vi "Compute Complementary Amplitude Multi-Exponential.vi"(8 "Error In":errorcluster, 9 "Time Constant Array":dbl[](array[numeric]), 11 "Amplitude Array":dbl[](array[numeric])) -> (0 "Error Out":errorcluster, 3 "Complementary Amplitude":dbl)   [LabVIEW 2021, in "Fits.lvlib"]
uses:
  Fits.lvlib
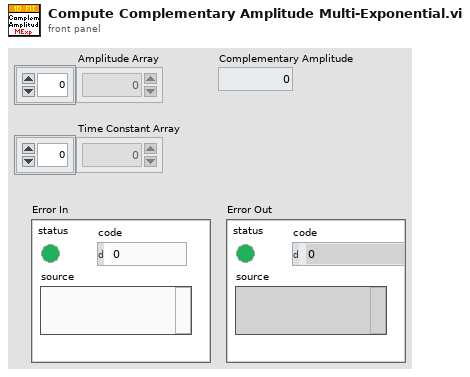
[diagram p1: front panel]
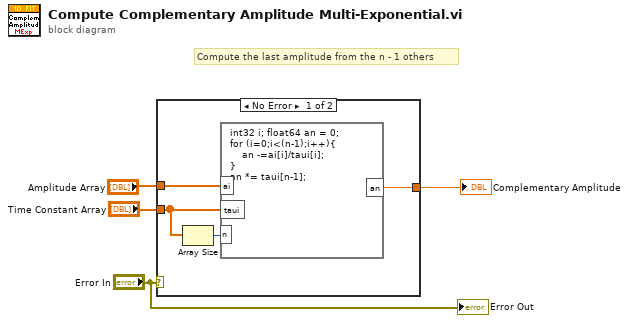
[diagram p0: block diagram]
diagram:
  # "Compute the last amplitude from the n - 1 others"
  n1 = case shown="No Error" "Error In" {
    tunnel: [w8 _] -> w4
    tunnel: "Amplitude Array" -> [w7 _]
    tunnel: "Time Constant Array" -> [w6 _]
    frame No Error {
      n2 = Array Size(array=w6) -> (size(s)=w5:i32)
      n3 = formula code="int32 i; float64 an = 0; \nfor (i=0;i<(n-1);i++){\n    an -=ai[i]/taui[i];\n}\nan *= taui[n-1];"("ai"=w7, "n"=w5, "taui"=w6) -> ("an"=w8:dbl)
    }
    frame Error {
    }
  }
  "Complementary Amplitude" <- w4
  "Error Out" <- "Error In"
